vi "Serie four.vi"() -> ()   [LabVIEW 2013]
panel:
  out "new picture":picture
  in  "L'ouverture de l'image":path
  in  "Valider":bool
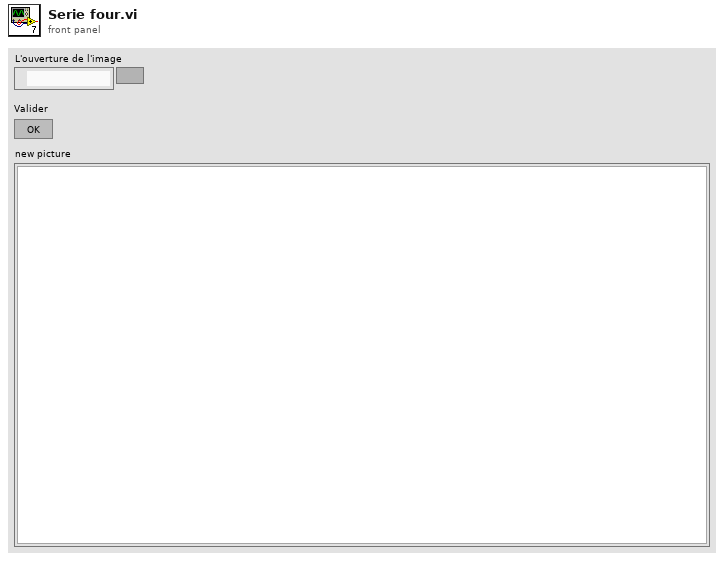
[diagram p1: front panel]
types:
  T1 = typedef "imagedata.ctl" = cluster{"image type":i32, "image depth":i32, "image":u8[], "mask":u8[], "colors":u32[], "Rectangle":cluster{"left":i16, "top":i16, "right":i16, "bottom":i16}}
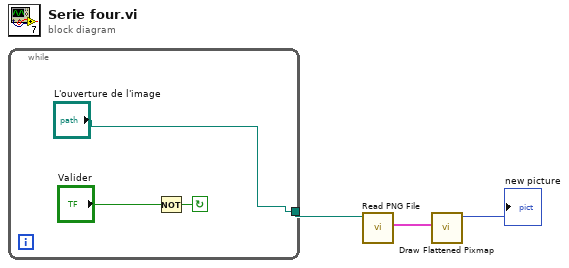
[diagram p0: block diagram]
diagram:
  n1 = while {
    tunnel: ["L'ouverture de l'image"] -> w3
    stop <- w4 continue-if-true
    n2 = Not(x="Valider") -> (.not. x?=w4:bool)
  }
  n3 = call <vilib>:"Read PNG File.vi"("path to PNG file"=w3) -> ("image data"=w2:T1)  [unwired: 8 in, 2 out]
  n4 = call <vilib>:"Draw Flattened Pixmap.vi"("image data"=w2) -> ("new picture"=→"new picture":picture)  [unwired: 8 in]
